vi "Offset Locking- Main with Slave Tracking v2.3.vi"() -> ()   [LabVIEW 2018]
uses:
  <vilib>/Utility/error.llb/DialogType.ctl
  <vilib>/Analysis/1siggen.llb/Ramp Pattern by Samples.vi
  <vilib>/measure/mamon.llb/Waveform Peak Detection for 1 Chan.vi
  <vilib>/addons/control/pid/pid.llb/PID Advanced (DBL).vi
  <vilib>/measure/NI_MAPro.lvlib
  <vilib>/addons/control/pid/NI_PID_pid.lvlib
  <vilib>/Analysis/NI_AALBase.lvlib
  <vilib>/measure/NI_MABase.lvlib
panel:
  in  "Slave Current Adjust":dbl(knob) scale=-10.0..10.0
  out "Target \nPeak":dbl
  out "Calibration\n Peaks":dbl[](array[numeric])
  in  "Minimum \namplitude\nfor Calibration":dbl=1.7 format="%#_13g V"
  in  "width":i32=1000
  in  "start":dbl format="%0.2f"
  in  "end":dbl=1.0 format="%0.2f"
  in  "samples":i32=128
  in  "Waveform Test?":bool
  in  "reset signal":bool
  in  "phase":dbl format="%.2p"
  out "Chirp Rate":dbl format="%#_g GHz/ms"
  out "Single Mode?":bool
  out "# of Peaks found when Chirping?":i32
  in  "Minimum amplitude for Slave":dbl=0.15 format="%.2p"
  in  "Minimum \namplitude\nfor peaks":dbl=0.6 format="%#_13g V"
  in  "PZT Voltage to \nFrequency Conversion":dbl=-1.41655 format="%#_g V/GHz"
  out "PZT Chirp Output":waveform(dbl)(graph)
  in  "offset":dbl format="%0.2p V"
  in  "Sampling Info":cluster{"Fs":dbl, "#s":dbl}={"Fs"=10000.0, "#s"=100.0} {"Fs" format="%.2p"}
  in  "frequency":dbl=10.0 format="%0.2p Hz"
  in  "Chirp Amplitude":dbl=1.5 format="%0.2p GHz"
  in  "Run Chirp Program?":bool
  out "Run Time (min)":dbl
  out "standard deviation":dbl format="%0.3e"
  out "# found":i32
  out "Offset":dbl(graph)
  in  "Manual PZT Control":dbl format="%#_g V"
  in  "Engage PZT PID?":bool
  out "Offset (GHz)":dbl format="%#_4g"
  in  "# of Shots for Averaging":i32=100
  in  "Name Convention":string="Chirp Offset Lock Log"
  in  "Save Directory":path=path "C:/Users/LabUser/Google Drive/Measurements/04-2018"
  out "Enough\n peaks?":bool
  out "PZT Output":dbl(graph)
  in  "PID Gains":T1={"proportional gain (Kc)"=-1.0, "integral time (Ti, min)"=0.01, "derivative time (Td, min)"=0.0} {"derivative time (Td, min)" format="%.3f"; "integral time (Ti, min)" format="%.3f"; "proportional gain (Kc)" format="%.3f"}
  out "dt out (s)":dbl format="%.3f"
  in  "Frequency Offset Setpoint (GHz)":dbl=4.0 format="%.3f"
  out "GHz/sec":dbl
  out "dt":dbl format="%#_4g"
  out "Locations":dbl[](array[numeric]) format="%.2p"
  out "Amplitudes":dbl[](array[numeric]) format="%.2p"
  out "2nd Derivatives":dbl[](array[numeric]) format="%.2p"
  out "10 GHz FPI":dynamicdata(graph)
  in  "Stop":bool
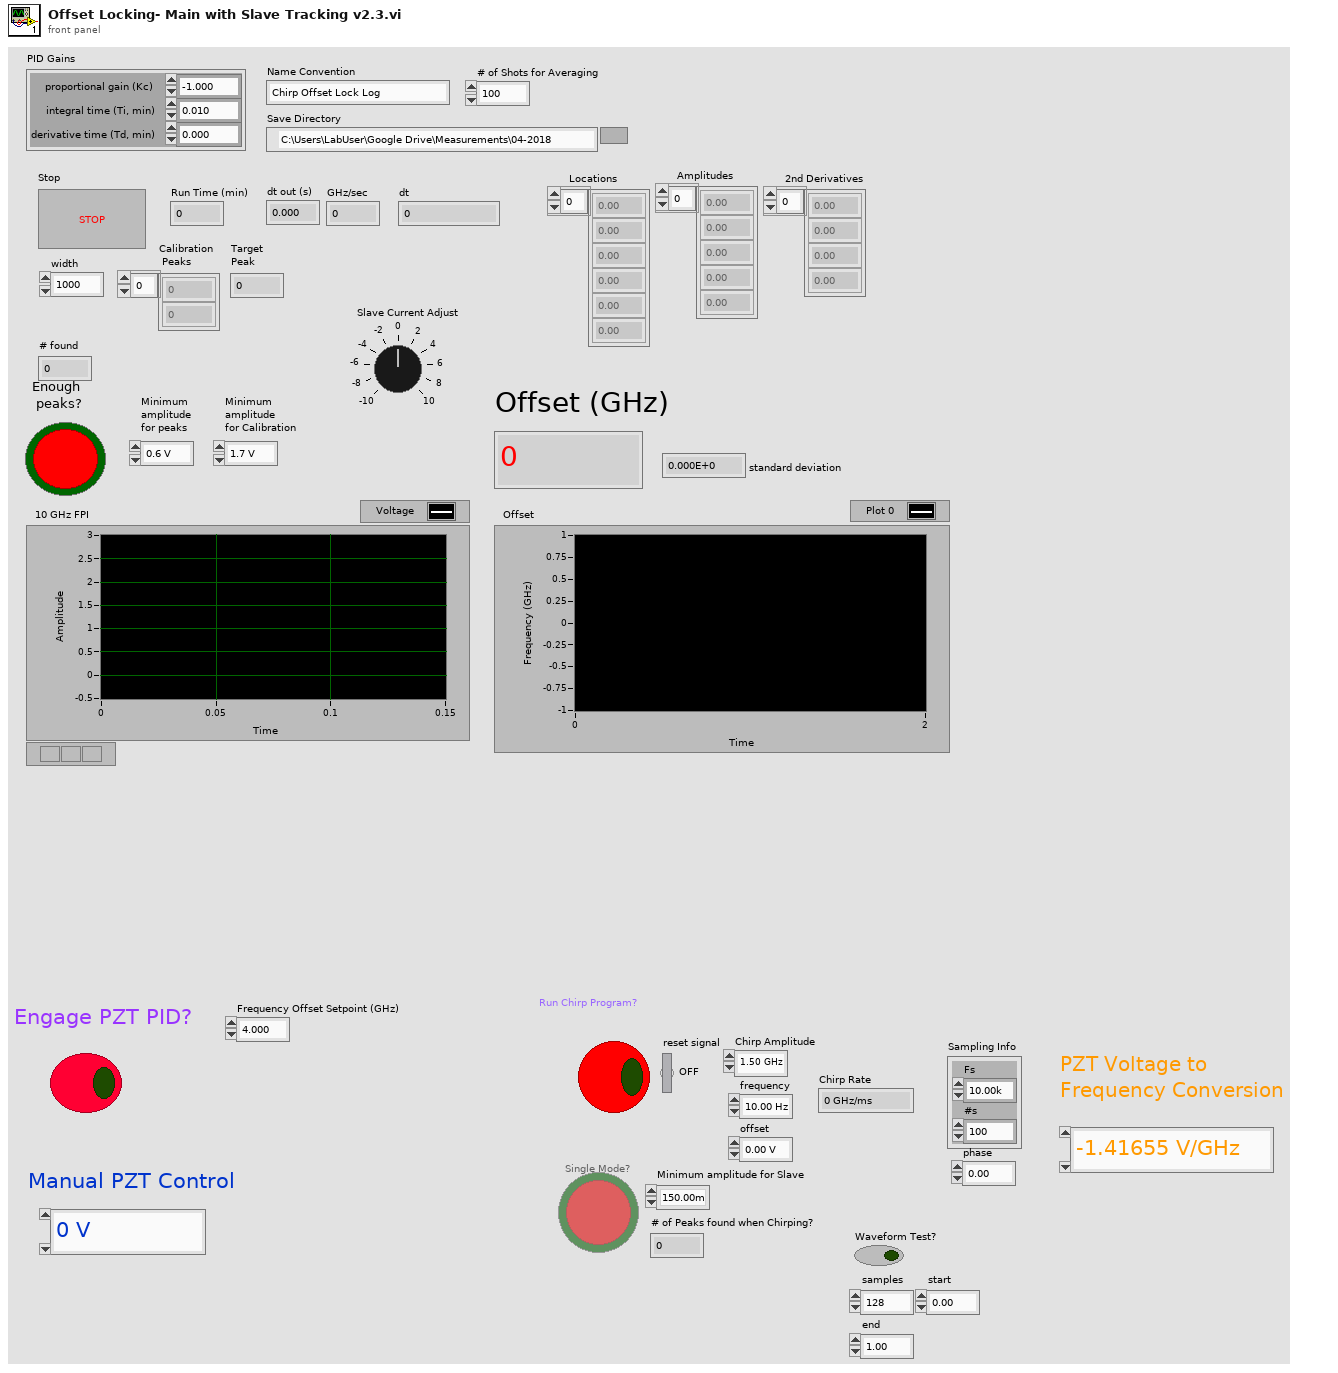
[diagram p1: front panel]
types:
  T1 = cluster{"proportional gain (Kc)":dbl, "integral time (Ti, min)":dbl, "derivative time (Td, min)":dbl}
  T2 = enum8{"Enabled", "Disabled", "Disabled and Grayed Out"}
  T3 = typedef "DialogType.ctl" = u16
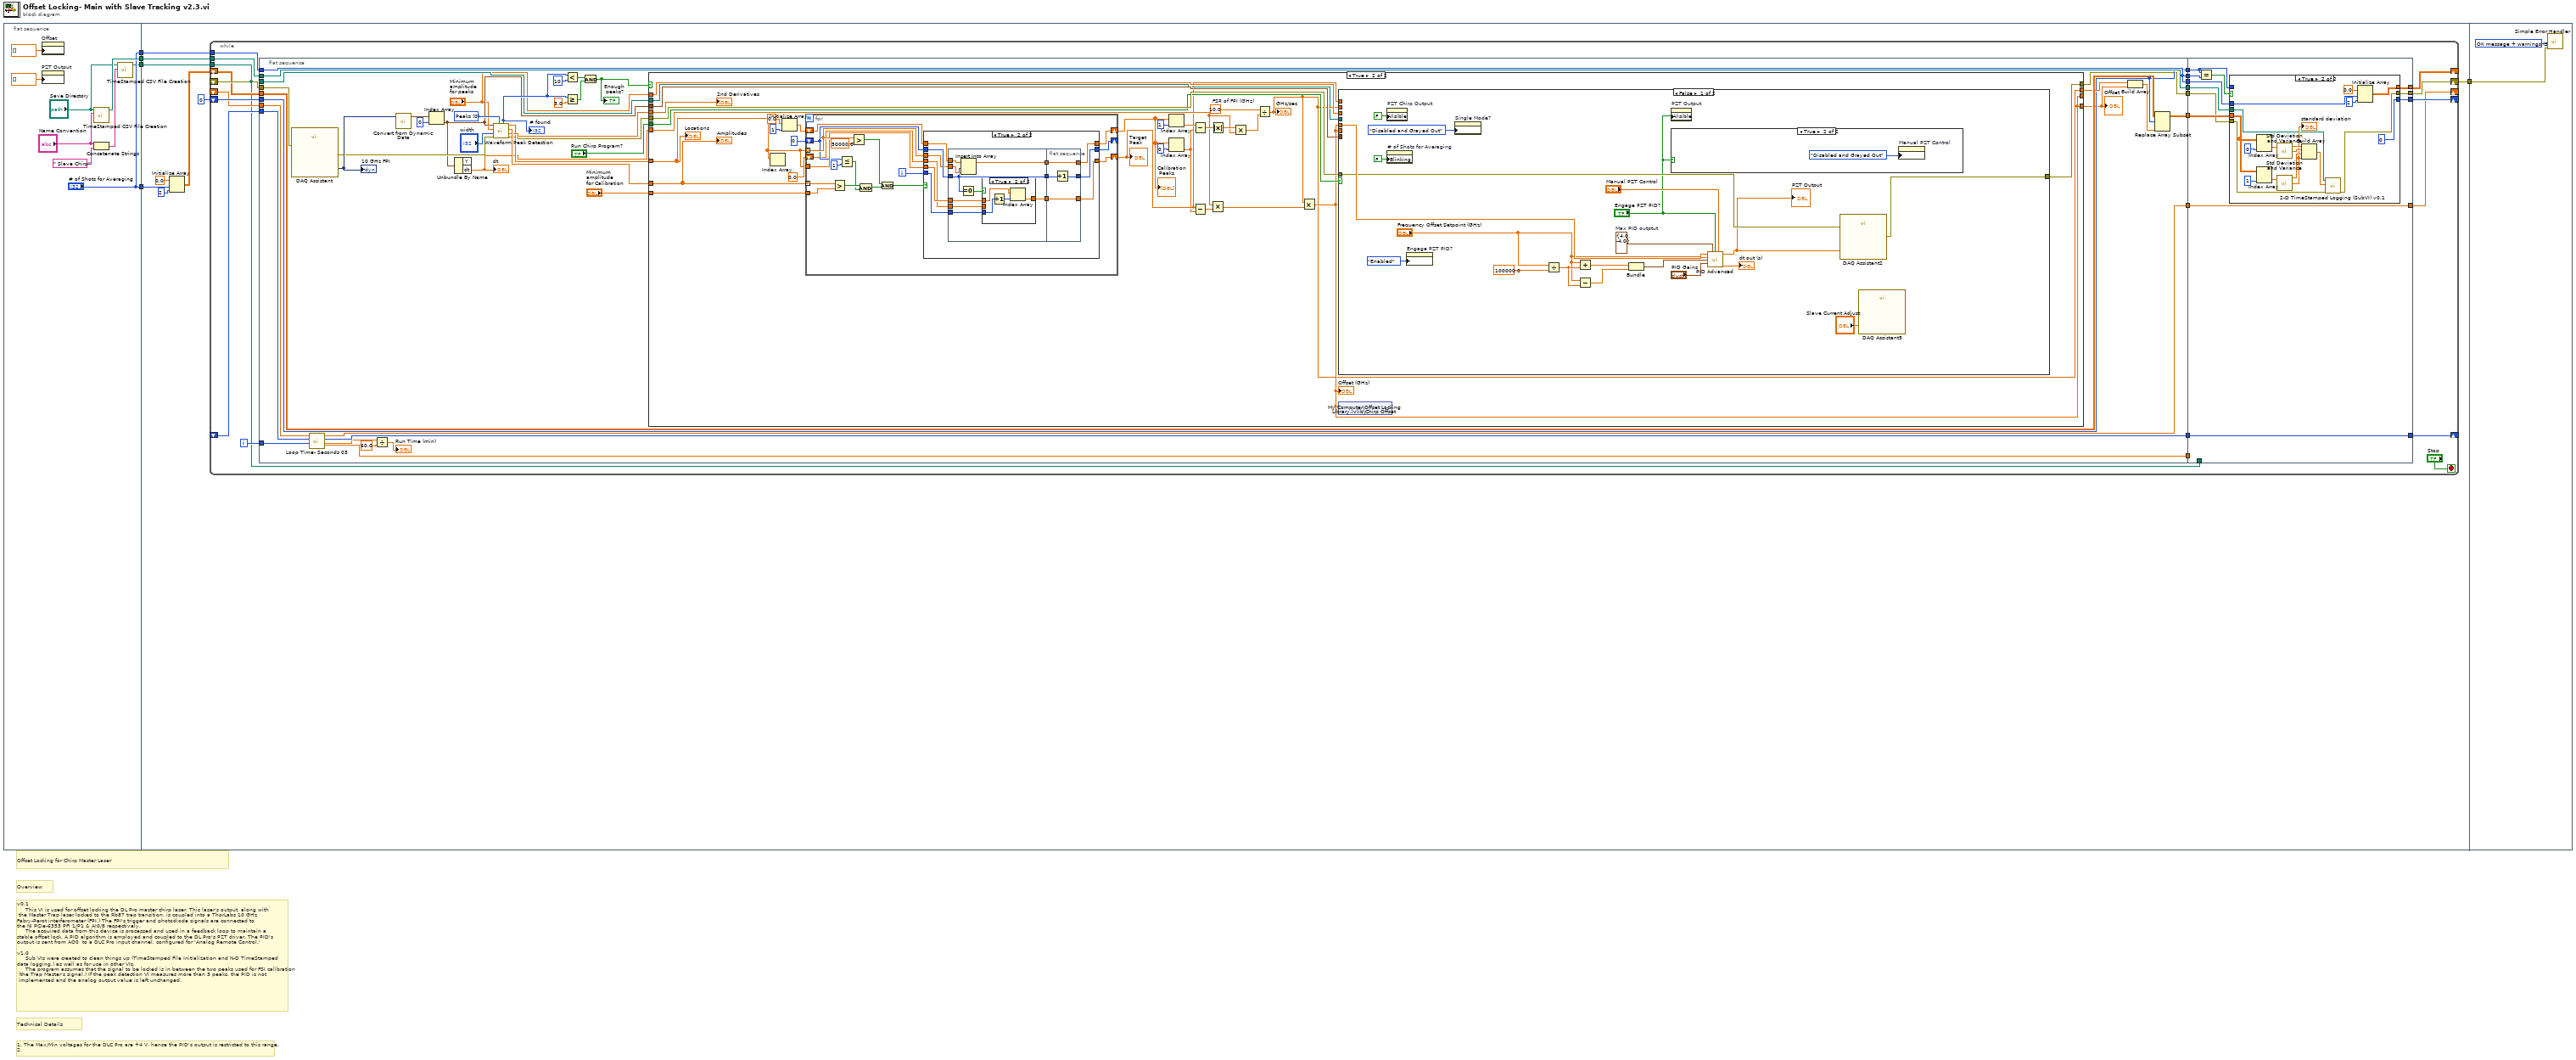
[diagram p0: block diagram]
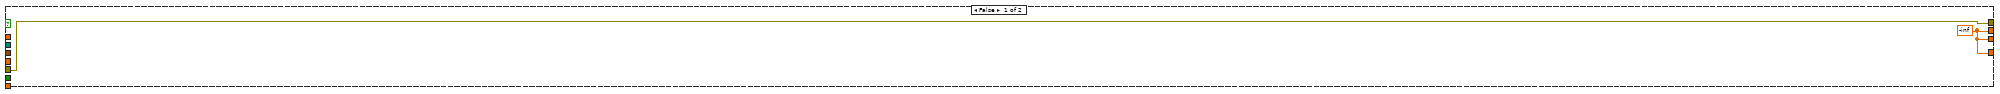
[diagram p2: hidden frame]
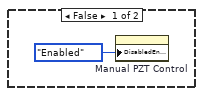
[diagram p5: hidden frame]
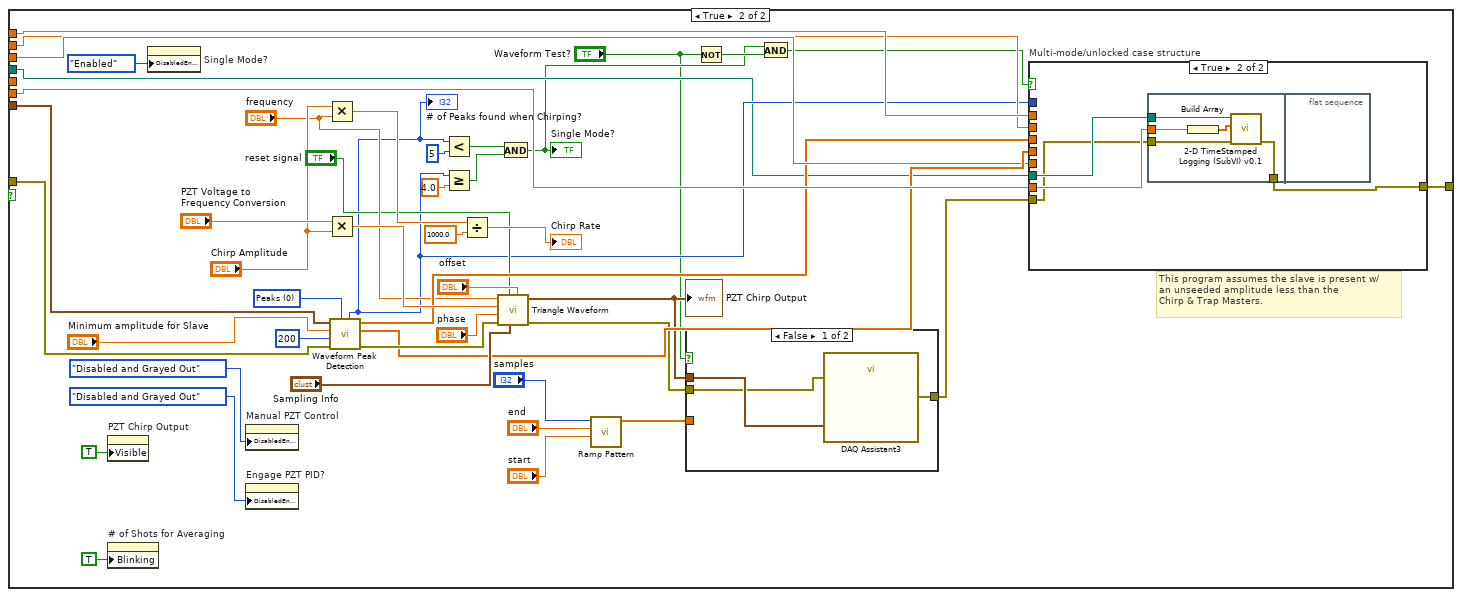
[diagram p6: hidden frame]
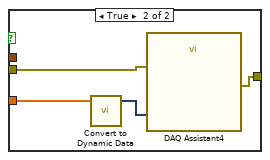
[diagram p7: hidden frame]
diagram:
  # "1. The Max/Min voltages for the DLC Pro are +4 V, hence the PID's output is restricted to this range.\n2."
  # "Technical Details"
  # "v0.1\n     This VI is used for offset locking the DL Pro master chirp laser. This laser's output, along with\n the Master Trap laser locked to the Rb87 trap transition, is coupled into a ThorLabs 10 GHz \nFabry-Perot interferometer (FPI.) The FPI's trigger and photodiode signals are connected to \nthe NI PCIe-6353 PFI 1/P1 & AI0/8 respectively. \n     The acquired data from this device is processed and used in a feedback loop to maintain a \nstable offset lock. A PID algorithm is employed and coupled to the DL Pro's PZT driver. The PID's\noutput is sent from AO0  to a DLC Pro input channel, configured for 'Analog Remote Control.'\n\nv1.0\n     Sub VIs were created to clean things up (TimeStamped File Initialization and N-D TimeStamped \ndata logging,) as well as for use in other VIs.\n     The program assumes that the signal to be locked is in between the two peaks used for FSI calibration\n (the Trap Master's signal.) If the peak detection VI measures more than 3 peaks, the PID is not\n implemented and the analog output value is left unchanged."
  # "Overview"
  # "Offset Locking for Chirp Master Laser"
  n1 = flat-sequence {
    tunnel: [w14] -> w5
    tunnel: ["# of Shots for Averaging"] -> w3
    tunnel: ["# of Shots for Averaging"] -> w2
    tunnel: [w6] -> w1
    tunnel: w5 -> [w23]
    tunnel: [w22] -> w4
    tunnel: w3 -> [w20]
    tunnel: w2 -> [w17]
    tunnel: w1 -> [w15]
    tunnel: w4 -> [w295]
    frame #0 {
      n2 = property on="Offset" class="WFChart (strict)"("History Data"=dbl[] []) -> ()  [unwired: 2 in, 2 out]
      n3 = property on="PZT Output" class="WFChart (strict)"("History Data"=dbl[] []) -> ()  [unwired: 2 in, 2 out]
      n4 = call "TimeStamped CSV File Creation.vi"("Name Convention"="Name Convention", "Save Directory"="Save Directory") -> ("path"=w14:path)  [unwired: 8 in, 1 out]
      n5 = Concatenate Strings("Name Convention", " Slave Chirp" ("string")) -> (w8:string)
      n6 = call "TimeStamped CSV File Creation.vi"("Name Convention"=w8, "Save Directory"="Save Directory") -> ("path"=w6:path)  [unwired: 8 in, 1 out]
    }
    frame #1 {
      n7 = Initialize Array(0.0 ("element"), w17, 2 ("dimension size")) -> (w19:dbl[][])
      n8 = while {
        shift-right: [w35] -> w22
        shift-left: _ -> [w46]
        tunnel: w23 -> [w44]
        shift-right: [w33] -> _
        shift-left: 0 -> [w42]
        tunnel: w20 -> [w40]
        shift-right: [w34] -> _
        shift-left: w19 -> [w37]
        shift-right: [w31] -> _
        shift-left: _ -> [w28]
        shift-right: [w29] -> _
        shift-left: _ -> [w27]
        tunnel: w15 -> [w24]
        i -> [w26]
        stop <- "Stop" stop-if-true
        n9 = flat-sequence {
          tunnel: w46 -> [w78]
          tunnel: [w54] -> w45
          tunnel: w44 -> [w76]
          tunnel: [w76] -> w43
          tunnel: w42 -> [w70]
          tunnel: [w70] -> w41
          tunnel: w40 -> [w71]
          tunnel: [w71] -> w39
          tunnel: [w75] -> w38
          tunnel: w37 -> [w74]
          tunnel: [w71] -> w36
          tunnel: [w69] -> w32
          tunnel: [w68] -> w30
          tunnel: w28 -> [w67]
          tunnel: w27 -> [w66]
          tunnel: w26 -> [w65]
          tunnel: [w57] -> w25
          tunnel: w24 -> [w51]
          tunnel: w45 -> [w268]
          tunnel: w43 -> [w269]
          tunnel: w41 -> [w263]
          tunnel: w39 -> [w273]
          tunnel: w38 -> [w270]
          tunnel: w36 -> [w271]
          tunnel: [w262] -> w35
          tunnel: [w267] -> w34
          tunnel: [w266] -> w33
          tunnel: w32 -> [w265]
          tunnel: [w265] -> w31
          tunnel: [w264] -> w29
          tunnel: w30 -> [w264]
          tunnel: w25 -> [_]
          tunnel: w24 -> [_]
          frame #0 {
            w80 = u16 0 items=["Peaks", "Valleys"] ("peaks/valleys")
            n10 = call "DAQ Assistant"("error in"=w78) -> ("data"=w85:dynamicdata, "error out"=w77:errorcluster)  [unwired: 16 in, 1 out]
            "10 GHz FPI" <- w85
            n11 = call "Loop Time- Seconds 03.vi"("Loop Iteration"=w65, "Shift Registered Time In"=w66, "Shift Registered In"=w67) -> ("t"=w57:dbl, "Shift Registered Time Out"=w68:u32, "Shift Registered Out"=w69:dbl)  [unwired: 6 in]
            n12 = Divide(x=w57, y=60.0) -> (x/y=→"Run Time (min)":dbl)
            n13 = call "Convert from Dynamic Data"("Dynamic Data Type"=w85) -> ("Array of Waveform"=w87:waveform(dbl)[])  [unwired: 3 in]
            n14 = Index Array(array=w87, index=0) -> (element=w52:waveform(dbl))
            n15 = Unbundle By Name(w52) -> ("dt"=w81:dbl)  [unwired: 1 out]
            "dt" <- w81
            n16 = call-poly <vilib>:"Waveform Peak Detection.vi"("peaks/valleys"=w80, "error in"=w77, "width"="width", "threshold"="Minimum \namplitude\nfor peaks", "Signal In"=w52) -> ("error out"=w55:errorcluster, "2nd Derivatives"=w83:dbl[], "Amplitudes"=w84:dbl[], "Locations"=w82:dbl[], "# found"=w62:i32)  [unwired: 2 in]
            "# found" <- w62
            n17 = Less?(x=w62, y=10) -> (x < y?=w60:bool)
            n18 = Greater Or Equal?(x=w62, y=3.0) -> (x >= y?=w63:bool)
            n19 = And(x=w60, y=w63) -> (x .and. y?=w59:bool)
            "Enough\n peaks?" <- w59
            n20 = case shown="True" w59 {
              tunnel: w84 -> [_ w103]
              tunnel: w83 -> [_ w119]
              tunnel: w82 -> [_ w96]
              tunnel: w81 -> [_ w113]
              tunnel: [w89 w105] -> w73
              tunnel: [w89 w107] -> w64
              tunnel: [w89 w107] -> _
              tunnel: w55 -> [w88 w111]
              tunnel: [w88 w110] -> w54
              tunnel: "Run Chirp Program?" -> [_ w109]
              tunnel: w52 -> [_ w108]
              tunnel: "Minimum \namplitude\nfor peaks" -> [_ w106]
              tunnel: w51 -> [_ w104]
              tunnel: "Minimum \namplitude\nfor Calibration" -> [_ w102]
              frame False {
                w89 = -inf
              }
              frame True {
                w118 = 10.0  # FSR of FPI (GHz)
                n21 = Index Array(array=w96) -> ()  [unwired: 1 in, 1 out]
                n22 = Initialize Array(0.0 ("element"), 1 ("dimension size")) -> (w98:dbl[])
                n23 = for {
                  tunnel: w96 -> [w126] mode=indexing
                  tunnel: w103 -> [w132] mode=indexing
                  tunnel: w102 -> [w131]
                  shift-right: [w122] -> w95
                  shift-left: w98 -> [w137]
                  shift-right: [w136] -> _
                  shift-left: 0 -> [w123]
                  shift-right: [w121] -> w91
                  shift-left: 0.0 -> [w120]
                  tunnel: w96 -> [w124]
                  i -> [w125]
                  n24 = Greater?(x=w132, y=w131) -> (0:w135:bool)
                  n25 = Less Or Equal?(x=w123, y=1) -> (x <= y?=w133:bool)
                  n26 = Greater?(x=w126, y=50000.0) -> (0:w129:bool)
                  n27 = And(x=w135, y=w133) -> (x .and. y?=w130:bool)
                  n28 = And(x=w129, y=w130) -> (x .and. y?=w127:bool)
                  n29 = case shown="True" w127 {
                    tunnel: w137 -> [w139 w152]
                    tunnel: w123 -> [w140 w151]
                    tunnel: [w140 w148] -> w136
                    tunnel: w126 -> [_ w150]
                    tunnel: w125 -> [_ w145]
                    tunnel: w124 -> [_ w144]
                    tunnel: [w139 w146] -> w122
                    tunnel: [w138 w142] -> w121
                    tunnel: w120 -> [w138 w141]
                    frame False {
                    }
                    frame True {
                      n30 = flat-sequence {
                        tunnel: w152 -> [w161]
                        tunnel: w151 -> [w158]
                        tunnel: w150 -> [w160]
                        tunnel: [w159] -> w149
                        tunnel: [w158] -> w147
                        tunnel: w145 -> [w155]
                        tunnel: w144 -> [w157]
                        tunnel: [w156] -> w143
                        tunnel: w141 -> [w153]
                        tunnel: w149 -> [w168]
                        tunnel: [w170] -> w148
                        tunnel: w147 -> [w169]
                        tunnel: [w168] -> w146
                        tunnel: w143 -> [w167]
                        tunnel: [w167] -> w142
                        frame #0 {
                          n31 = Equal To 0?(x=w158) -> (x = 0?=w154:bool)
                          n32 = Insert Into Array(array=w161, index=w158, new element=w160) -> (w159:dbl[])
                          n33 = case shown="True" w154 {
                            tunnel: w157 -> [_ w166]
                            tunnel: [w162 w165] -> w156
                            tunnel: w155 -> [_ w163]
                            tunnel: w153 -> [w162 _]
                            frame False {
                            }
                            frame True {
                              n34 = Increment(x=w163) -> (x+1=w164:i32)
                              n35 = Index Array(array=w166, index=w164) -> (element=w165:dbl)
                            }
                          }
                        }
                        frame #1 {
                          n36 = Increment(x=w169) -> (x+1=w170:i32)
                        }
                      }
                    }
                  }
                }
                "Calibration\n Peaks" <- w95
                "Target \nPeak" <- w91
                n37 = Index Array(array=w95, index=1) -> (element=w92:dbl)
                n38 = Index Array(array=w95, index=0) -> (element=w90:dbl)
                n39 = Subtract(x=w92, y=w90) -> (x-y=w116:dbl)
                n40 = Subtract(x=w91, y=w90) -> (x-y=w114:dbl)
                n41 = Multiply(x=w113, y=w114) -> (x*y=w112:dbl)
                n42 = Absolute Value(x=w116) -> (abs(x)=w115:dbl)
                n43 = Multiply(x=w115, y=w113) -> (x*y=w117:dbl)
                n44 = Divide(x=w118, y=w117) -> (x/y=w105:dbl)
                "GHz/sec" <- w105
                n45 = Multiply(x=w105, y=w112) -> (x*y=w107:dbl)
                "Offset (GHz)" <- w107
                n46 = case shown="False" w109 {
                  tunnel: w107 -> [w186 _]
                  tunnel: w111 -> [w185 w228]
                  tunnel: [w184 w201] -> w110
                  tunnel: w108 -> [_ w229]
                  tunnel: w107 -> [_ w225]
                  tunnel: w106 -> [_ w219]
                  tunnel: w91 -> [_ w217]
                  tunnel: w105 -> [_ w216]
                  tunnel: w104 -> [_ w203]
                  frame False {
                    w188 = cluster{"output high":dbl, "output low":dbl} {"output high"=4.0, "output low"=-4.0}  # Max PID outptut
                    n47 = property on="PZT Chirp Output" class="WFGraph (strict)"("Visible"=FALSE) -> ()  [unwired: 2 in, 2 out]
                    n48 = property on="# of Shots for Averaging" class="DigNum (strict)"("Blinking"=FALSE) -> ()  [unwired: 2 in, 2 out]
                    n49 = property on="Engage PZT PID?" class="Bool (strict)"("DisabledEnum"=T2."Enabled" ("Disabled")) -> ()  [unwired: 2 in, 2 out]
                    n50 = property on="Single Mode?" class="Bool (strict)"("DisabledEnum"=T2."Disabled and Grayed Out" ("Disabled")) -> ()  [unwired: 2 in, 2 out]
                    n51 = Divide(x="Frequency Offset Setpoint (GHz)", y=100000.0) -> (x/y=w176:dbl)
                    n52 = Add(x="Frequency Offset Setpoint (GHz)", y=w176) -> (x+y=w174:dbl)
                    n53 = Subtract(x="Frequency Offset Setpoint (GHz)", y=w176) -> (x-y=w173:dbl)
                    n54 = Bundle(w174, w173) -> (w172:cluster{dbl, dbl})  [unwired: 1 in]
                    n55 = property on="PZT Output" class="WFChart (strict)"("Visible"="Engage PZT PID?") -> ()  [unwired: 2 in, 2 out]
                    n56 = case shown="True" "Engage PZT PID?" {
                      frame False {
                        n57 = property on="Manual PZT Control" class="DigNum (strict)"("DisabledEnum"=T2."Enabled" ("Disabled")) -> ()  [unwired: 2 in, 2 out]
                      }
                      frame True {
                        n58 = property on="Manual PZT Control" class="DigNum (strict)"("DisabledEnum"=T2."Disabled and Grayed Out" ("Disabled")) -> ()  [unwired: 2 in, 2 out]
                      }
                    }
                    n59 = call-poly <vilib>:"PID Advanced.vi"("setpoint"="Frequency Offset Setpoint (GHz)", "output range"=w188, "auto? (T)"="Engage PZT PID?", "manual control"="Manual PZT Control", "process variable"=w186, "setpoint range"=w172, "PID gains"="PID Gains") -> ("output"=w183:dbl, "dt out (s)"=→"dt out (s)":dbl)  [unwired: 7 in]
                    "PZT Output" <- w183
                    n60 = call "DAQ Assistant2"("data"=w183, "error in"=w185) -> ("error out"=w184:errorcluster)  [unwired: 16 in, 1 out]
                    n61 = call "DAQ Assistant5"("data"="Slave Current Adjust") -> ()  [unwired: 17 in, 2 out]
                  }
                  frame True {
                    w215 = u16 0 items=["Peaks", "Valleys"] ("peaks/valleys")
                    # "This program assumes the slave is present w/ \nan unseeded amplitude less than the \nChirp & Trap Masters."
                    n62 = property on="PZT Chirp Output" class="WFGraph (strict)"("Visible"=TRUE) -> ()  [unwired: 2 in, 2 out]
                    n63 = property on="# of Shots for Averaging" class="DigNum (strict)"("Blinking"=TRUE) -> ()  [unwired: 2 in, 2 out]
                    n64 = property on="Single Mode?" class="Bool (strict)"("DisabledEnum"=T2."Enabled" ("Disabled")) -> ()  [unwired: 2 in, 2 out]
                    n65 = property on="Manual PZT Control" class="DigNum (strict)"("DisabledEnum"=T2."Disabled and Grayed Out" ("Disabled")) -> ()  [unwired: 2 in, 2 out]
                    n66 = property on="Engage PZT PID?" class="Bool (strict)"("DisabledEnum"=T2."Disabled and Grayed Out" ("Disabled")) -> ()  [unwired: 2 in, 2 out]
                    n67 = Multiply(x="Chirp Amplitude", y="frequency") -> (x*y=w210:dbl)
                    n68 = Multiply(x="PZT Voltage to \nFrequency Conversion", y="Chirp Amplitude") -> (x*y=w231:dbl)
                    n69 = call-poly <vilib>:"Waveform Peak Detection.vi"("peaks/valleys"=w215, "error in"=w228, "width"=200, "threshold"="Minimum amplitude for Slave", "Signal In"=w229) -> ("error out"=w227:errorcluster, "Amplitudes"=w220:dbl[], "Locations"=w218:dbl[], "# found"=w204:i32)  [unwired: 2 in, 1 out]
                    "# of Peaks found when Chirping?" <- w204
                    n70 = Less?(x=w204, y=5) -> (x < y?=w221:bool)
                    n71 = Greater Or Equal?(x=w204, y=4.0) -> (x >= y?=w223:bool)
                    n72 = Divide(x=w210, y=1000.0) -> (x/y=→"Chirp Rate":dbl)
                    n73 = call <vilib>:"Triangle Waveform.vi"("offset"="offset", "sampling info"="Sampling Info", "reset signal"="reset signal", "error in (no error)"=w227, "phase"="phase", "amplitude"=w231, "frequency"="frequency") -> ("error out"=w205:errorcluster, "signal out"=w206:waveform(dbl))  [unwired: 3 in]
                    "PZT Chirp Output" <- w206
                    n74 = And(x=w221, y=w223) -> (x .and. y?=w199:bool)
                    "Single Mode?" <- w199
                    n75 = call-poly <vilib>:"Ramp Pattern.vi"("start"="start", "end"="end", "samples"="samples") -> ("Ramp Pattern"=w196:dbl[])  [unwired: 7 in, 1 out]
                    n76 = case shown="False" "Waveform Test?" {
                      tunnel: w206 -> [w241 _]
                      tunnel: w205 -> [w240 w245]
                      tunnel: [w239 w244] -> w202
                      tunnel: w196 -> [_ w243]
                      frame False {
                        n77 = call "DAQ Assistant3"("data"=w241, "error in"=w240) -> ("error out"=w239:errorcluster)  [unwired: 16 in, 1 out]
                      }
                      frame True {
                        n78 = call "Convert to Dynamic Data"("Array"=w243) -> ("Dynamic Data Type"=w242:dynamicdata)  [unwired: 3 in]
                        n79 = call "DAQ Assistant4"("data"=w242, "error in"=w245) -> ("error out"=w244:errorcluster)  [unwired: 16 in, 1 out]
                      }
                    }
                    n80 = Not(x="Waveform Test?") -> (.not. x?=w200:bool)
                    n81 = And(x=w199, y=w200) -> (x .and. y?=w198:bool)
                    n82 = case "Multi-mode/unlocked case structure" shown="True" w198 {
                      tunnel: w225 -> [_ w256]
                      tunnel: w204 -> [w252 _]
                      tunnel: w220 -> [w251 _]
                      tunnel: w219 -> [w250 _]
                      tunnel: w218 -> [w249 _]
                      tunnel: w217 -> [w248 _]
                      tunnel: w216 -> [w247 _]
                      tunnel: w203 -> [_ w255]
                      tunnel: w202 -> [w246 w254]
                      tunnel: [w246 w253] -> w201
                      frame False {
                        n83 = for {
                          N: w252 -> [_]
                          tunnel: w251 -> [_] mode=indexing
                          tunnel: w250 -> [_]
                          tunnel: w249 -> [_] mode=indexing
                          tunnel: w248 -> [_]
                          tunnel: w247 -> [_]
                        }
                      }
                      frame True {
                        n84 = flat-sequence {
                          tunnel: w256 -> [w261]
                          tunnel: w255 -> [w259]
                          tunnel: w254 -> [w258]
                          tunnel: [w257] -> w253
                          frame #0 {
                            n85 = Build Array(w261) -> (w260:dbl[])
                            n86 = call "2-D TimeStamped Logging (SubVI) v0.1.vi"("error in (no error)"=w258, "array"=w260, "path"=w259) -> ("error out"=w257:errorcluster)  [unwired: 8 in]
                          }
                          frame #1 {
                          }
                        }
                      }
                    }
                  }
                }
                n87 = shared-variable "My Computer\\Offset Locking Library.lvlib\\Chirp Offset"(w107) -> ()  [unwired: 1 in, 1 out]
                "2nd Derivatives" <- w119
                "Amplitudes" <- w103
                "Locations" <- w96
              }
            }
            "Offset" <- w64
            n88 = Build Array(w73, w64) -> (w72:dbl[])
            n89 = Replace Array Subset(array=w74, new element=w72, index (row)=w70) -> (w75:dbl[][])  [unwired: 1 in]
          }
          frame #1 {
            n90 = Equal?(x=w263, y=w273) -> (x = y?=w272:bool)
            n91 = case shown="True" w272 {
              tunnel: w271 -> [_ w277]
              tunnel: w270 -> [w276 w290]
              tunnel: w269 -> [_ w284]
              tunnel: w268 -> [w274 w283]
              tunnel: [w276 w280] -> w267
              tunnel: w263 -> [w275 _]
              tunnel: [w275 0] -> w266
              tunnel: [w274 w278] -> w262
              frame False {
              }
              frame True {
                n92 = Index Array(array=w290, index (col)=0 ("disabled index (col)")) -> (element=w293:dbl[])  [unwired: 1 in]
                n93 = Index Array(array=w290, index (col)=1 ("disabled index (col)")) -> (element=w291:dbl[])  [unwired: 1 in]
                n94 = call <vilib>:"Std Deviation and Variance.vi"("X"=w293) -> ("mean"=w289:dbl, "standard deviation"=w288:dbl)  [unwired: 1 in, 1 out]
                n95 = call <vilib>:"Std Deviation and Variance.vi"("X"=w291) -> ("mean"=w287:dbl, "standard deviation"=w286:dbl)  [unwired: 1 in, 1 out]
                "standard deviation" <- w286
                n96 = Build Array(w289, w288, w287, w286) -> (w285:dbl[])
                n97 = call "2-D TimeStamped Logging (SubVI) v0.1.vi"("error in (no error)"=w283, "array"=w285, "path"=w284) -> ("error out"=w278:errorcluster)  [unwired: 8 in]
                n98 = Initialize Array(0.0 ("element"), w277, 2 ("dimension size")) -> (w280:dbl[][])
              }
            }
          }
        }
      }
    }
    frame #2 {
      w296 = T3 3 items=["no dialog", "OK message", "continue or stop message", "OK message + warnings", "continue/stop + warnings"] ("type of dialog (OK msg:1)")
      n99 = call <vilib>:"Simple Error Handler.vi"("type of dialog (OK msg:1)"=w296, "error in (no error)"=w295) -> ()  [unwired: 3 in, 5 out]
    }
  }
